vi "Create Frame Pattern Script.vi"(8 "error in (no error)":errorcluster, 10 "SPI_FRM_Config":T1 {"Addr" format="%x"; "Data" format="%x"}, 11 "SPI_Frame_Read_Collect in":refnum<class "SPI_Frame_Read_Collect.lvclass">) -> (0 "error out":errorcluster, 3 "SPI_Frame_Read_Collect out":refnum<class "SPI_Frame_Read_Collect.lvclass">)   [LabVIEW 2018, in "SPI_Frame_Read_Collect.lvclass"]
uses:
  SPI_Frame_Read_Collect.lvclass
  C:/P4 Workspace/PC Client/Solutions/5g_eap/HiSi/trunk/1.0/BML_Pattern_Gen_Refactor/SPI/SPI Frame Root/SPI_Frame_Root.lvclass
  Config Read SPI/SPI_FRM_Config.ctl
  Classes/Config_Read/RW_Option.ctl
  Config Read SPI/SPI_Mode.ctl
  Classes/BML_Frame_Root/Special Frame.ctl
  SPI Frame Root/DataType.ctl
  SPI Frame Root/SPI_Frame_Root.lvclass/SPI_Frame_Root.ctl
  Classes/BML_Frame_Root/BML_Frame_Root.lvclass
  SPI Frame Root/SPI_Frame_Root.lvclass
  Classes/Config_Read/Config_Read_BML.lvclass
  Config Read SPI/Config_Read_SPI.lvclass
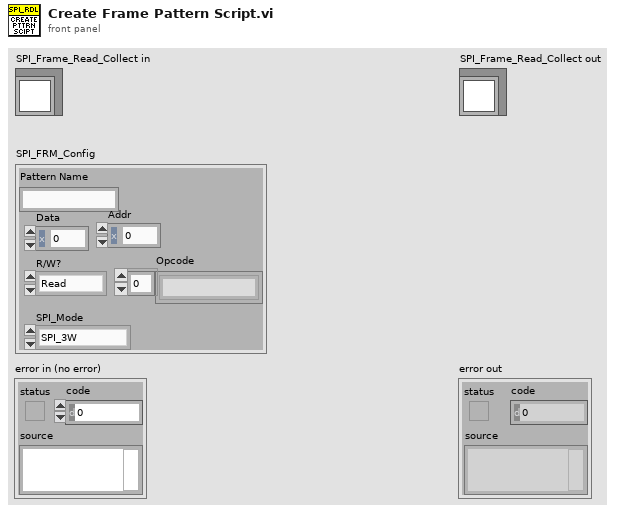
[diagram p1: front panel]
types:
  T1 = typedef "Config_Read_SPI.lvclass/SPI_FRM_Config.ctl" = cluster{"Pattern Name":string, "Data":u16, "Addr":u16, "R/W?":T2, "Opcode":string[], "SPI_Mode":T3}
  T2 = typedef "Config_Read_BML.lvclass/RW_Option.ctl" = enum16{"Read", "Write", "R/W"}
  T3 = typedef "Config_Read_SPI.lvclass/SPI_Mode.ctl" = enum16{"SPI_3W", "SPI_4W"}
  T4 = typedef "BML_Frame_Root.lvclass/Special Frame.ctl" = enum16{"Sync Header", "Protocol Header", "SW Trig", "SetID State", "Out SetID State", "SW Reset", "Wait", "SPI 4W FRM Start", "SPI 4W Wait", "SPI 4W FRM End", "SPI 4W Write Cmd", "SPI RD Collect Cmd", "SPI RD Value Cmd", "SPI 3W FRM Start", "SPI 3W Write Cmd", "SPI 3W FRM End", "SPI 3W Wait", "SPI 3W RD Cmd"}
  T5 = typedef "SPI_Frame_Root.lvclass/DataType.ctl" = enum16{"Drive", "Compare", "Read"}
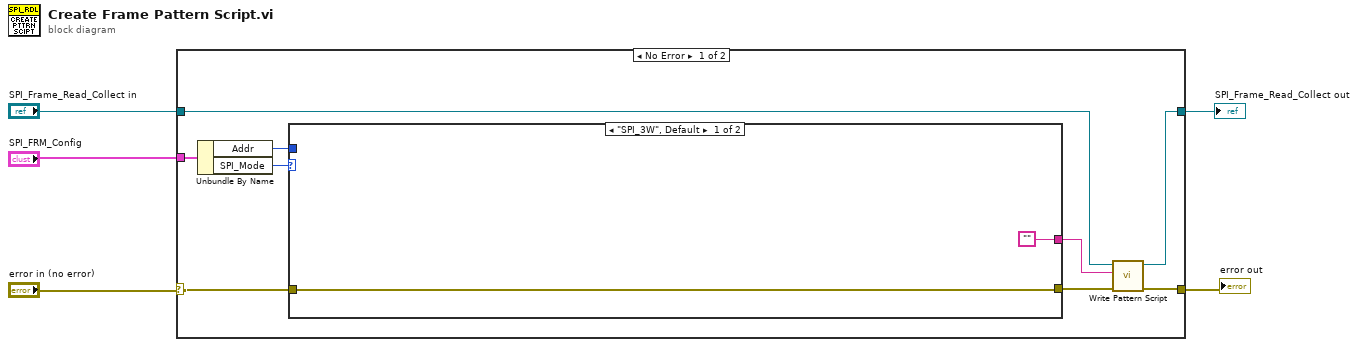
[diagram p0: block diagram]
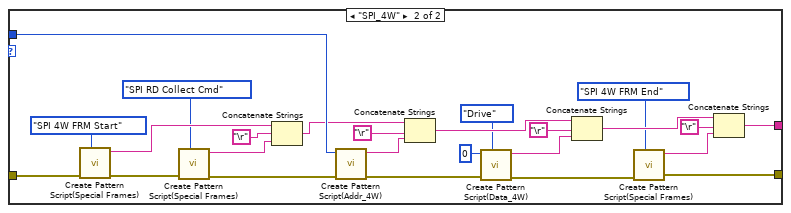
[diagram p2: hidden frame]
diagram:
  n1 = case shown="No Error" "error in (no error)" {
    selector: "error in (no error)" -> [w11 w42]
    tunnel: [w7 w43] -> w3
    tunnel: "SPI_Frame_Read_Collect in" -> [w8 w43]
    tunnel: [w10 w42] -> w2
    tunnel: "SPI_FRM_Config" -> [w9 _]
    frame No Error {
      n2 = Unbundle By Name(w9) -> ("Addr"=w14:u16, "SPI_Mode"=w6:T3)
      n3 = case shown="\"SPI_3W\", Default" w6 {
        tunnel: w14 -> [_ w41]
        tunnel: [w16 w22] -> w13
        tunnel: ["" w21] -> w12
        tunnel: w11 -> [w16 w20]
        frame "SPI_3W", Default {
        }
        frame "SPI_4W" {
          n4 = call "Create Pattern Script(Special Frames).vi"("Special Frame Type"=Special_Frame."SPI 4W FRM Start", "error in (no error)"=w20) -> ("error out"=w27:errorcluster, "string out"=w29:string)  [unwired: 8 in]
          n5 = call "Create Pattern Script(Special Frames).vi"("Special Frame Type"=Special_Frame."SPI RD Collect Cmd", "error in (no error)"=w27) -> ("error out"=w32:errorcluster, "string out"=w31:string)  [unwired: 8 in]
          n6 = Concatenate Strings(w29, "\r", w31) -> (w33:string)
          n7 = call "Create Pattern Script(Addr_4W).vi"("error in (no error)"=w32, "Addr"=w41) -> ("error out"=w36:errorcluster, "String"=w35:string)  [unwired: 8 in]
          n8 = Concatenate Strings(w33, "\r", w35) -> (w38:string)
          n9 = call "Create Pattern Script(Data_4W).vi"("DataType"=DataType."Drive", "error in (no error)"=w36, "Data"=u16 0) -> ("error out"=w26:errorcluster, "String"=w40:string)  [unwired: 7 in]
          n10 = Concatenate Strings(w38, "\r", w40) -> (w25:string)
          n11 = call "Create Pattern Script(Special Frames).vi"("Special Frame Type"=Special_Frame."SPI 4W FRM End", "error in (no error)"=w26) -> ("error out"=w22:errorcluster, "string out"=w23:string)  [unwired: 8 in]
          n12 = Concatenate Strings(w25, "\r", w23) -> (w21:string)
        }
      }
      n13 = call "Write Pattern Script.vi"("error in (no error)"=w13, "Pattern Script"=w12, "SPI_Frame_Root in"=w8) -> ("error out"=w10:errorcluster, "SPI_Frame_Root out"=w7:refnum<class "SPI_Frame_Read_Collect.lvclass">)  [unwired: 7 in]
    }
    frame Error {
    }
  }
  "error out" <- w2
  "SPI_Frame_Read_Collect out" <- w3
